vi "8-dist.vi"(0 "n":u16) -> (1 "R rg médian":dbl[](array[numeric]), 2 "Rangs":i32[](array[numeric]))   [LabVIEW 2010, in "lv_02.lvlib"]
uses:
  lv_02.lvlib
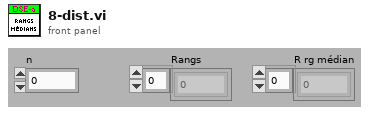
[diagram p1: front panel]
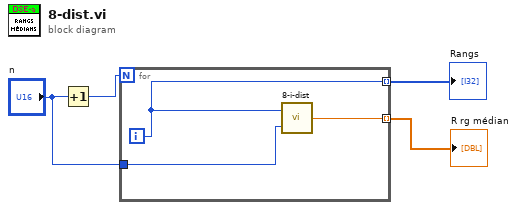
[diagram p0: block diagram]
diagram:
  n1 = Increment(x="n") -> (x+1=w4:u16)
  n2 = for {
    N: w4 -> [_]
    tunnel: [w6] -> w3 mode=indexing
    tunnel: [w7] -> w2 mode=indexing
    tunnel: "n" -> [w5]
    i -> [w7]
    n3 = call "8-i-dist.vi"("n"=w5, "i"=w7) -> ("R(i) médian obs_n"=w6:dbl)
  }
  "R rg médian" <- w3
  "Rangs" <- w2
